vi "Test Timer.vi"() -> ()   [LabVIEW 2012]
uses:
  Type Defs/Alt Control.ctl
  Type Defs/Alt Digit 100 New.ctl
panel:
  out "Elapsed Time (s)":dbl
  in  "Confirm Now 2":bool
  in  "ALT SET 2":T1 {"Alt Digit 100" min=0 max=9 step=1; "Alt Digit 100" min=0 max=9 step=1; "Alt Digit 100" min=0 max=9 step=1; "Alt Digit 100" min=0 max=9 step=1; "Alt Digit 100" min=0 max=9 step=1}
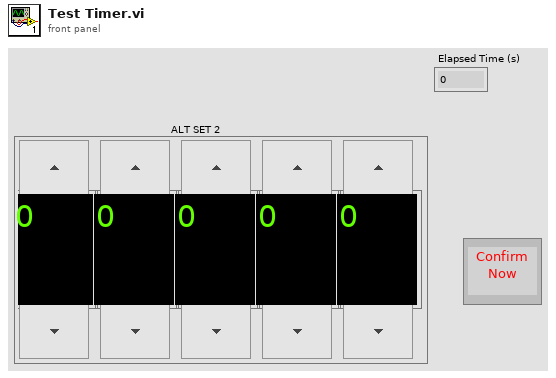
[diagram p1: front panel]
types:
  T1 = typedef "Alt Control.ctl" = cluster{"Alt Digit 100":T2, "Alt Digit 100":T2, "Alt Digit 100":T2, "Alt Digit 100":T2, "Alt Digit 100":T2}
  T2 = typedef "Alt Digit 100 New.ctl" = i8
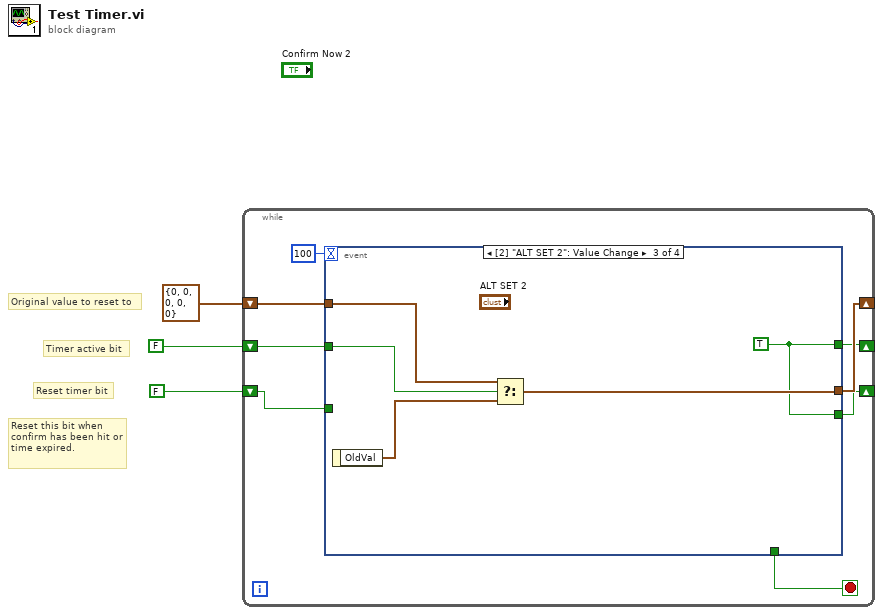
[diagram p0: block diagram]
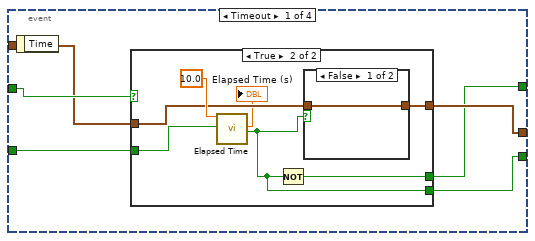
[diagram p2: hidden frame]
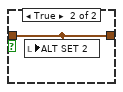
[diagram p4: hidden frame]
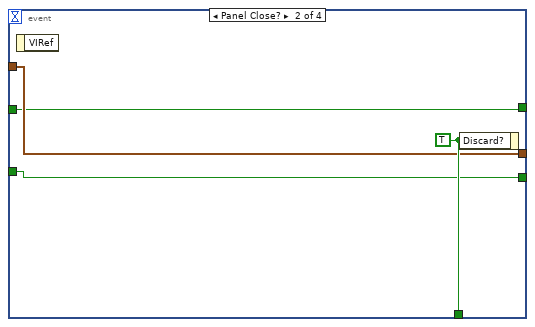
[diagram p5: hidden frame]
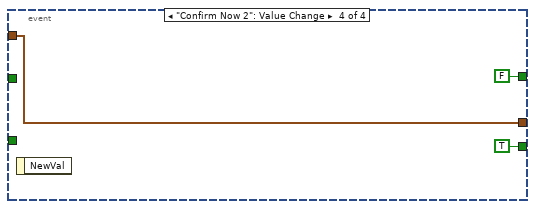
[diagram p6: hidden frame]
diagram:
  # "Original value to reset to"
  # "Timer active bit"
  # "Reset timer bit"
  # "Reset this bit when confirm has been hit or time expired."
  n1 = while {
    shift-right: [w7] -> _
    shift-left: T1 {"Alt Digit 100"=0, "Alt Digit 100"=0, "Alt Digit 100"=0, "Alt Digit 100"=0, "Alt Digit 100"=0} ("ALT SET 2") -> [w8]
    shift-right: [w6] -> _
    shift-left: FALSE -> [w9]
    shift-right: [w5] -> _
    shift-left: FALSE -> [w4]
    stop <- w11 stop-if-true
    n2 = event shown="[2] \"ALT SET 2\": Value Change" {
      selector: _ -> [_ _ _ _]
      dyn-events: _ -> [_ _ _ _]
      timeout: 100 -> [_ _ _ _]
      tunnel: [_ w33 _ _] -> w11
      tunnel: w9 -> [w17 w31 w38 _]
      tunnel: w8 -> [w15 w32 w37 w40]
      tunnel: [w14 w32 w35 w40] -> w7
      tunnel: [w13 w31 w34 FALSE] -> w6
      tunnel: [w12 w30 w34 TRUE] -> w5
      tunnel: w4 -> [w16 w30 _ _]
      event Timeout {
        n3 = event-data() -> ()  [unwired: 1 in, 1 out]
        n4 = case shown="True" w17 {
          selector: w17 -> [w18 _]
          tunnel: w16 -> [w19 w27]
          tunnel: w15 -> [w20 w25]
          tunnel: [w20 w24] -> w14
          tunnel: [w18 w23] -> w13
          tunnel: [w19 w22] -> w12
          frame False {
          }
          frame True {
            n5 = call "Elapsed Time"("Time Target (s)"=10.0, "Reset"=w27) -> ("Elapsed Time (s)"=→"Elapsed Time (s)":dbl, "Time has Elapsed"=w22:bool)  [unwired: 10 in, 6 out]
            n6 = Not(x=w22) -> (.not. x?=w23:bool)
            n7 = case shown="False" w22 {
              tunnel: w25 -> [w28 w29]
              tunnel: [w28 w29] -> w24
              frame False {
              }
              frame True {
                n8 = local write "ALT SET 2"(w29) -> ()
              }
            }
          }
        }
      }
      event Panel Close? {
        w33 = TRUE ("Discard?")
        n9 = event-data() -> ()  [unwired: 1 in, 1 out]
        n10 = event-data("Discard?"=w33) -> ()  [unwired: 1 in, 1 out]
      }
      event Value Change {
        w34 = TRUE
        n11 = event-data() -> ("OldVal"=w36:T1)  [unwired: 1 in]
        n12 = Select(t=w37, s=w38, f=w36) -> (s? t:f=w35:T1)
      }
      event "Confirm Now 2": Value Change {
        n13 = event-data() -> ()  [unwired: 1 in, 1 out]
      }
    }
  }
